vi "Validate Measurment Configurations.vi"(8 "error in":errorcluster, 11 "measurement configuration in":T1) -> (0 "error out":errorcluster, 2 "Waveforms":waveform(dbl)[](array[waveform]), 3 "measurement configuration out":T1)   [LabVIEW 2025, in "Fgen Script Mode.lvclass"]
uses:
  Fgen Script Mode.lvclass
  <vilib>/ErrorRing/Error Ring.xnode
  Fgen Script Mode.lvclass/Fgen Script Mode.ctl
  <vilib>/Utility/error.llb/Error Cluster From Error Code.vi
  Typedef/Wfm Typedef.ctl
  Measurement Configuration.ctl
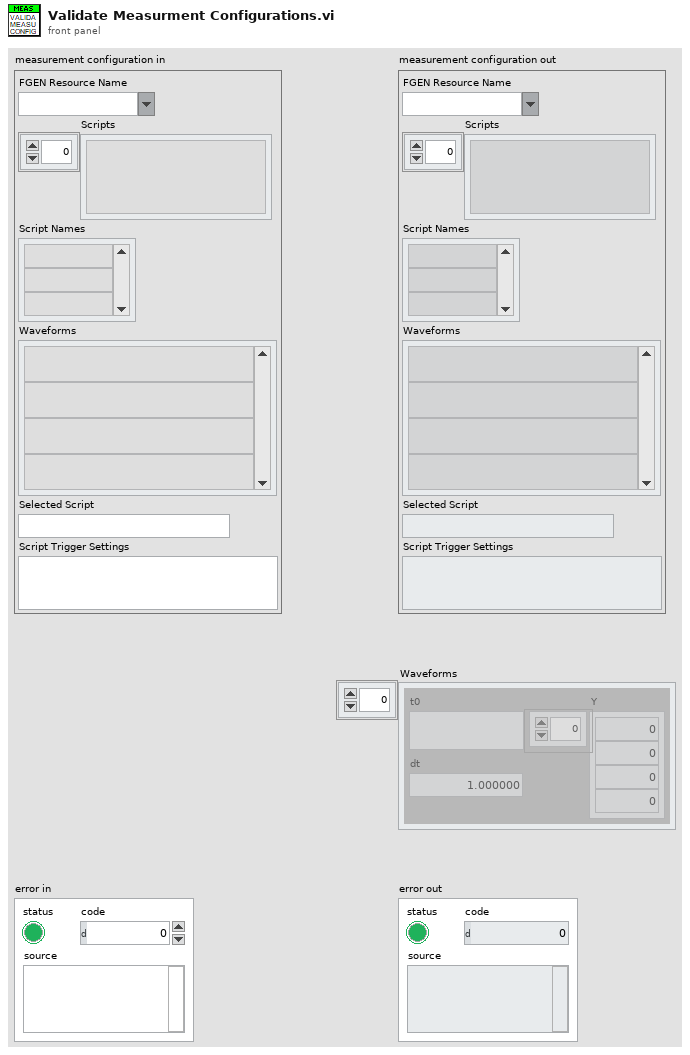
[diagram p1: front panel]
types:
  T1 = typedef "Fgen Script Mode.lvclass/Measurement Configuration.ctl" = cluster{"FGEN Resource Name":string, "Scripts":string[], "Script Names":string[], "Waveforms":string[], "Selected Script":string, "Script Trigger Settings":string}
  T2 = typedef "Fgen Script Mode.lvclass/Wfm Typedef.ctl" = cluster{"Name":string, "Path":string, "Grp":string, "Chn":string}
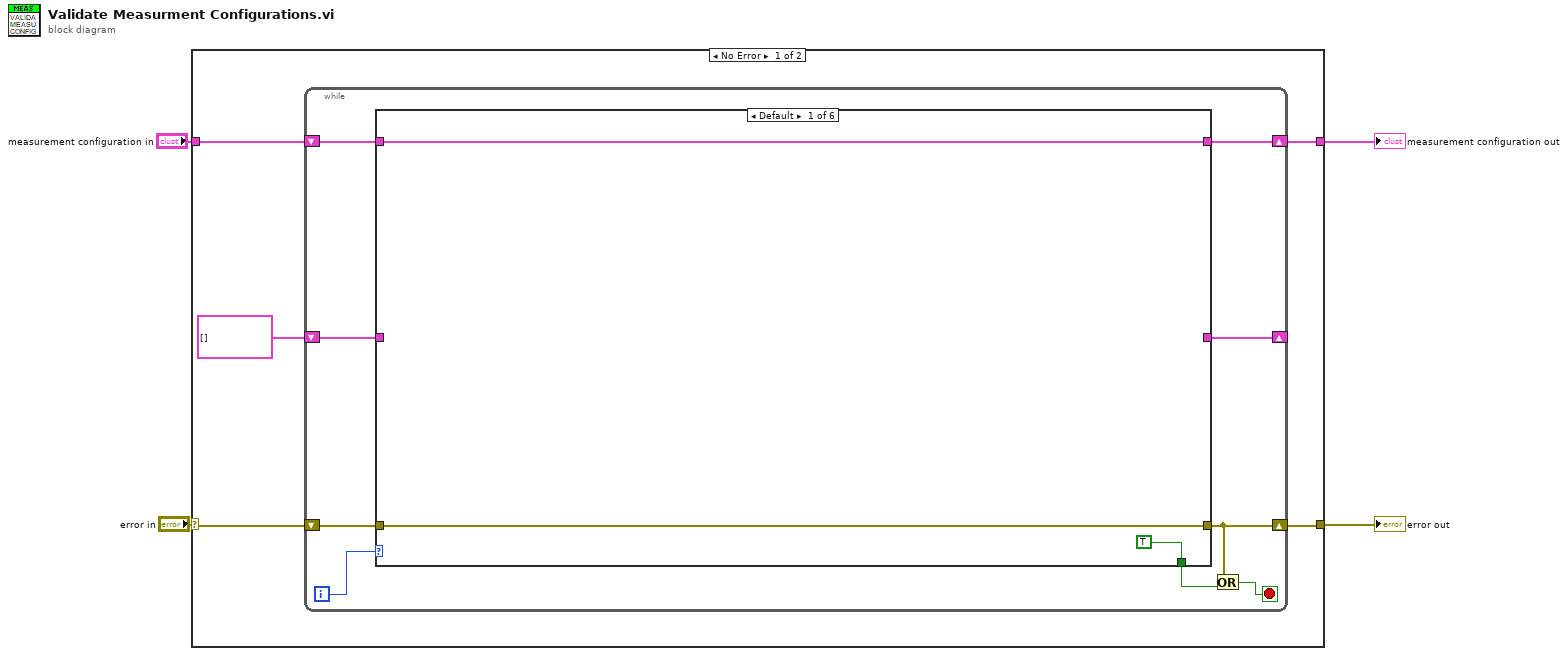
[diagram p0: block diagram]
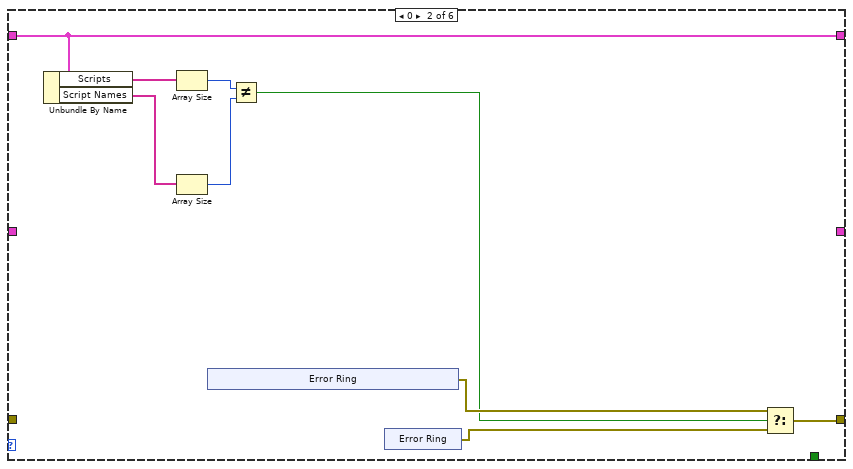
[diagram p2: hidden frame]
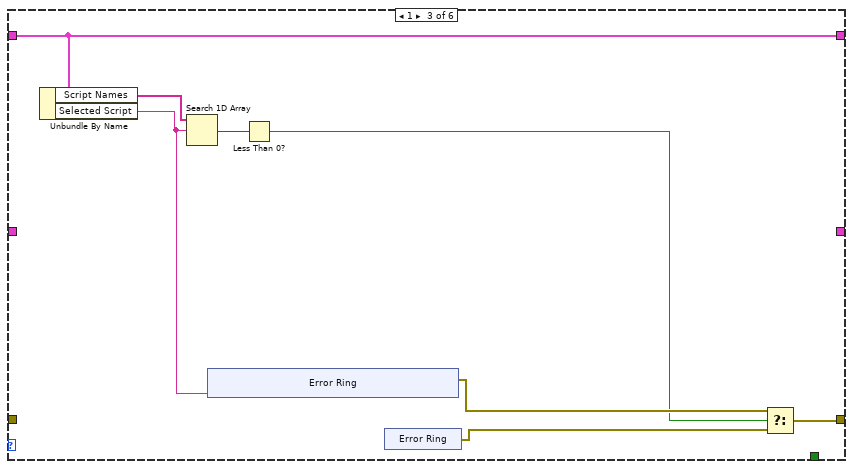
[diagram p3: hidden frame]
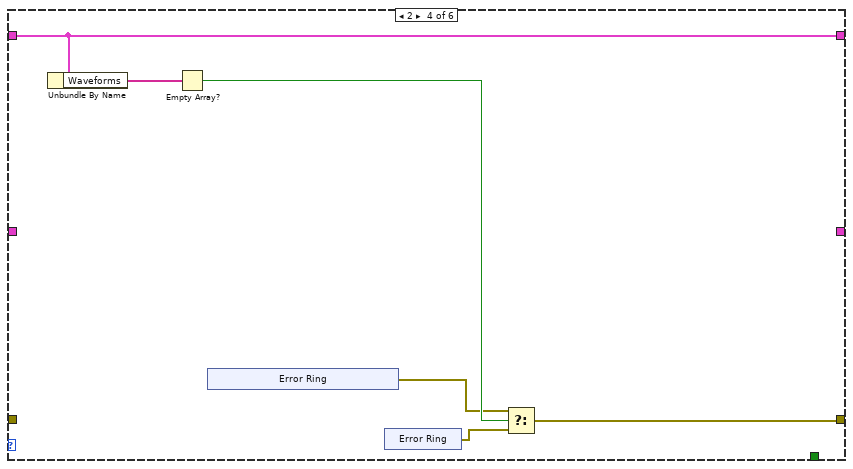
[diagram p4: hidden frame]
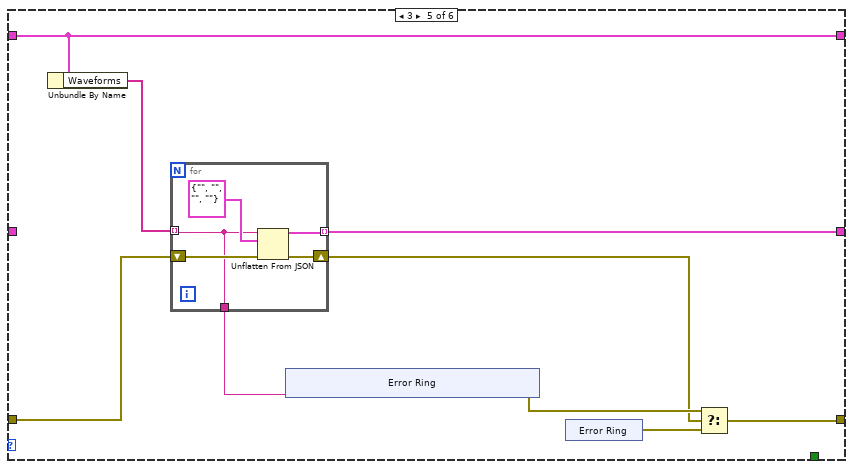
[diagram p5: hidden frame]
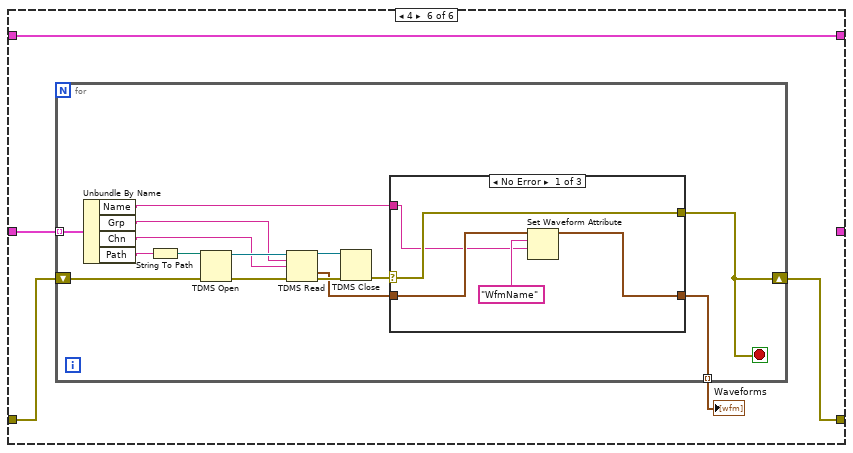
[diagram p6: hidden frame]
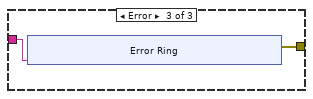
[diagram p8: hidden frame]
diagram:
  n1 = case shown="No Error" "error in" {
    selector: "error in" -> [w6 w123]
    tunnel: [w7 w123] -> w3
    tunnel: "measurement configuration in" -> [w9 w122]
    tunnel: [w8 w122] -> w1
    frame No Error {
      n2 = while {
        shift-right: [w16] -> w8
        shift-left: w9 -> [w17]
        shift-right: [w15] -> w7
        shift-left: w6 -> [w14]
        shift-right: [w13] -> _
        shift-left: T2[] [] -> [w12]
        i -> [w18]
        stop <- w11 stop-if-true
        n3 = case shown="Default" w18 {
          tunnel: w17 -> [w21 w30 w44 w58 w73 w91]
          tunnel: [w21 w30 w44 w58 w73 w91] -> w16
          tunnel: [w20 w22 w41 w53 w70 w88] -> w15
          tunnel: w14 -> [w20 _ _ _ w68 w89]
          tunnel: [_ _ _ _ w66 _] -> w13
          tunnel: w12 -> [_ _ _ _ _ w90]
          tunnel: [TRUE _ _ _ _ _] -> w10
          frame Default {
          }
          frame 0 {
            n4 = Unbundle By Name(w30) -> ("Scripts"=w29:string[], "Script Names"=w28:string[])
            n5 = Array Size(array=w29) -> (size(s)=w26:i32)
            n6 = Array Size(array=w28) -> (size(s)=w27:i32)
            n7 = xnode "Error Ring"() -> ("error out"=w24:errorcluster)
            n8 = Not Equal?(x=w26, y=w27) -> (x != y?=w23:bool)
            n9 = xnode "Error Ring"() -> ("error out"=w25:errorcluster)
            n10 = Select(t=w24, s=w23, f=w25) -> (s? t:f=w22:errorcluster)
          }
          frame 1 {
            n11 = Unbundle By Name(w44) -> ("Script Names"=w40:string[], "Selected Script"=w37:string)
            n12 = Search 1D Array(1D array=w40, element=w37) -> (index of element=w39:i32)  [unwired: 1 in]
            n13 = xnode "Error Ring"("parameter 0"=w37) -> ("error out"=w42:errorcluster)
            n14 = Less Than 0?(x=w39) -> (x < 0?=w38:bool)
            n15 = xnode "Error Ring"() -> ("error out"=w43:errorcluster)
            n16 = Select(t=w42, s=w38, f=w43) -> (s? t:f=w41:errorcluster)
          }
          frame 2 {
            n17 = Unbundle By Name(w58) -> ("Waveforms"=w57:string[])
            n18 = Empty Array?(array=w57) -> (empty?=w56:bool)
            n19 = xnode "Error Ring"() -> ("error out"=w54:errorcluster)
            n20 = xnode "Error Ring"() -> ("error out"=w55:errorcluster)
            n21 = Select(t=w54, s=w56, f=w55) -> (s? t:f=w53:errorcluster)
          }
          frame 3 {
            n22 = Unbundle By Name(w73) -> ("Waveforms"=w69:string[])
            n23 = for {
              tunnel: w69 -> [w74] mode=indexing
              shift-right: [w77] -> w67
              shift-left: w68 -> [w76]
              tunnel: [w75] -> w66 mode=indexing
              tunnel: [w74] -> w65
              n24 = Unflatten From JSON(JSON string=w74, type and defaults=T2 {"Name"="", "Path"="", "Grp"="", "Chn"=""} ("Waveform"), error in (no error)=w76) -> (value=w75:T2, error out=w77:errorcluster)  [unwired: 4 in]
            }
            n25 = xnode "Error Ring"("parameter 0"=w65) -> ("error out"=w71:errorcluster)
            n26 = xnode "Error Ring"() -> ("error out"=w72:errorcluster)
            n27 = Select(t=w71, s=w67, f=w72) -> (s? t:f=w70:errorcluster)
          }
          frame 4 {
            n28 = for {
              tunnel: w90 -> [w106] mode=indexing
              shift-right: [w93] -> w88
              shift-left: w89 -> [w94]
              tunnel: [w92] -> w87 mode=indexing
              stop <- w93 stop-if-true
              n29 = Unbundle By Name(w106) -> ("Name"=w98:string, "Grp"=w97:string, "Chn"=w96:string, "Path"=w95:string)
              n30 = String To Path(string=w95) -> (path=w105:path)
              n31 = TDMS Open(8:w94, 11:w105) -> (0:w103:errorcluster, 3:w104:refnum<k34>)  [unwired: 5 in]
              n32 = TDMS Read(0:w104, 5:w97, 7:w96, 11:w103) -> (4:w101:refnum<k34>, 10:w99:waveform(dbl), 15:w102:errorcluster)  [unwired: 4 in, 3 out]
              n33 = TDMS Close(8:w102, 11:w101) -> (0:w100:errorcluster)  [unwired: 1 out]
              n34 = case shown="No Error" w100 {
                selector: w100 -> [w111 w112 _]
                tunnel: [w111 w112 w114] -> w93
                tunnel: w99 -> [w110 _ _]
                tunnel: [w109 _ _] -> w92
                tunnel: w98 -> [w107 _ w113]
                frame No Error {
                  n35 = Set Waveform Attribute(5:w107, 6:"WfmName" ("name"), 7:w110) -> (3:w109:waveform(dbl))  [unwired: 1 in, 2 out]
                }
                frame Default {
                }
                frame Error {
                  n36 = xnode "Error Ring"("parameter 0"=w113) -> ("error out"=w114:errorcluster)
                }
              }
            }
            "Waveforms" <- w87
          }
        }
        n37 = Or(x=w15, y=w10) -> (x .or. y?=w11:bool)
      }
    }
    frame Error {
    }
  }
  "measurement configuration out" <- w1
  "error out" <- w3
